vi "Launch Staff Manager.vi"(0 "Hotel Management Tool Model in":refnum<class "Hotel Management Tool Model.lvclass">, 11 "error in (no error)":errorcluster) -> (4 "Hotel Management Tool Model out":refnum<class "Hotel Management Tool Model.lvclass">, 15 "error out":errorcluster)   [LabVIEW 2023, in "Hotel Management Tool Model.lvlib" / "Hotel Management Tool Model.lvclass"]
uses:
  Hotel Management Tool Model.lvclass
  Staff Manager Model/Staff Manager Model/Staff Manager Model.lvclass
  Hotel Management Tool Model.lvclass/Hotel Management Tool Model.ctl
  <vilib>/ActorFramework/Actor/Actor.lvclass
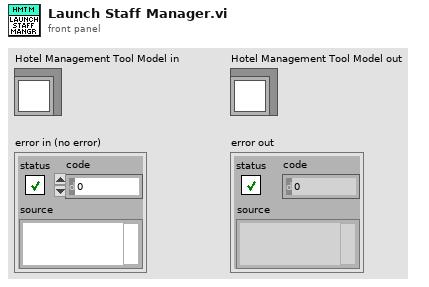
[diagram p1: front panel]
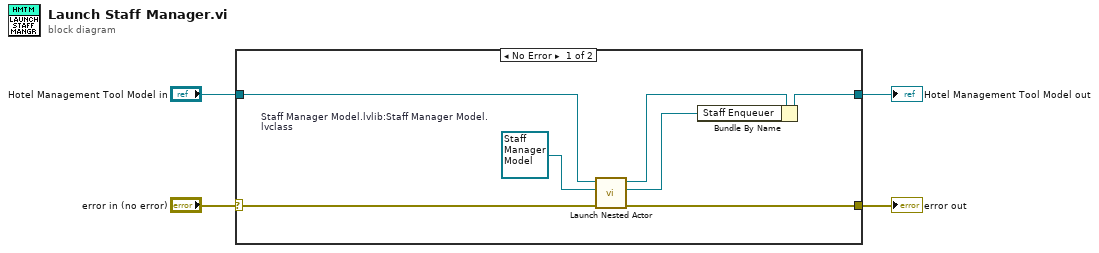
[diagram p0: block diagram]
diagram:
  n1 = case shown="No Error" "error in (no error)" {
    selector: "error in (no error)" -> [w11 w13]
    tunnel: [w10 w13] -> w1
    tunnel: [w7 w12] -> w2
    tunnel: "Hotel Management Tool Model in" -> [w9 w12]
    frame No Error {
      w5 = refnum<class "Staff Manager Model.lvclass"> refnum  # Staff Manager Model.lvlib:Staff Manager Model.lvclass
      n2 = call <vilib>:"Launch Nested Actor.vi"("error in (no error)"=w11, "Nested Actor"=w5, "Caller Actor in"=w9) -> ("error out"=w10:errorcluster, "Nested Actor's Enqueuer"=w6:refnum<class "Message Enqueuer.lvclass">, "Caller Actor out"=w8:refnum<class "Hotel Management Tool Model.lvclass">)  [unwired: 6 in]
      n3 = Bundle By Name(cluster=w8, "Staff Enqueuer"=w6) -> (w7:refnum<class "Hotel Management Tool Model.lvclass">)
    }
    frame Error {
    }
  }
  "error out" <- w1
  "Hotel Management Tool Model out" <- w2
